vi "LV_multiports_multiservers.vi"() -> ()   [LabVIEW 2020]
panel:
  out "2nd port":string
  out "1st port":string
  in  "Open Multi Ports":bool
  in  "Send Test Img":bool
  in  "h":i32=10 min=1 max=5000 step=1
  in  "w":i32=1 min=1 max=5000 step=1
  out "Elaps ms":u32
  in  "Send Image":bool
  out "Path to Python script":path
  in  "Stop":bool
  out "Answer":string
  in  "Ping":bool
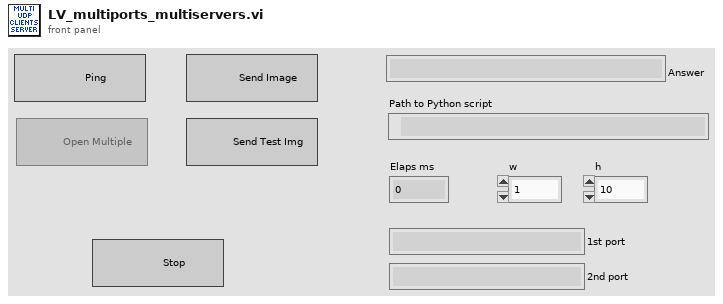
[diagram p1: front panel]
types:
  T1 = enum8{"Enabled", "Disabled", "Disabled and Grayed Out"}
  T2 = typedef "Image Type" = u32
  T3 = typedef "IMAQ Image.ctl" = refnum<image>
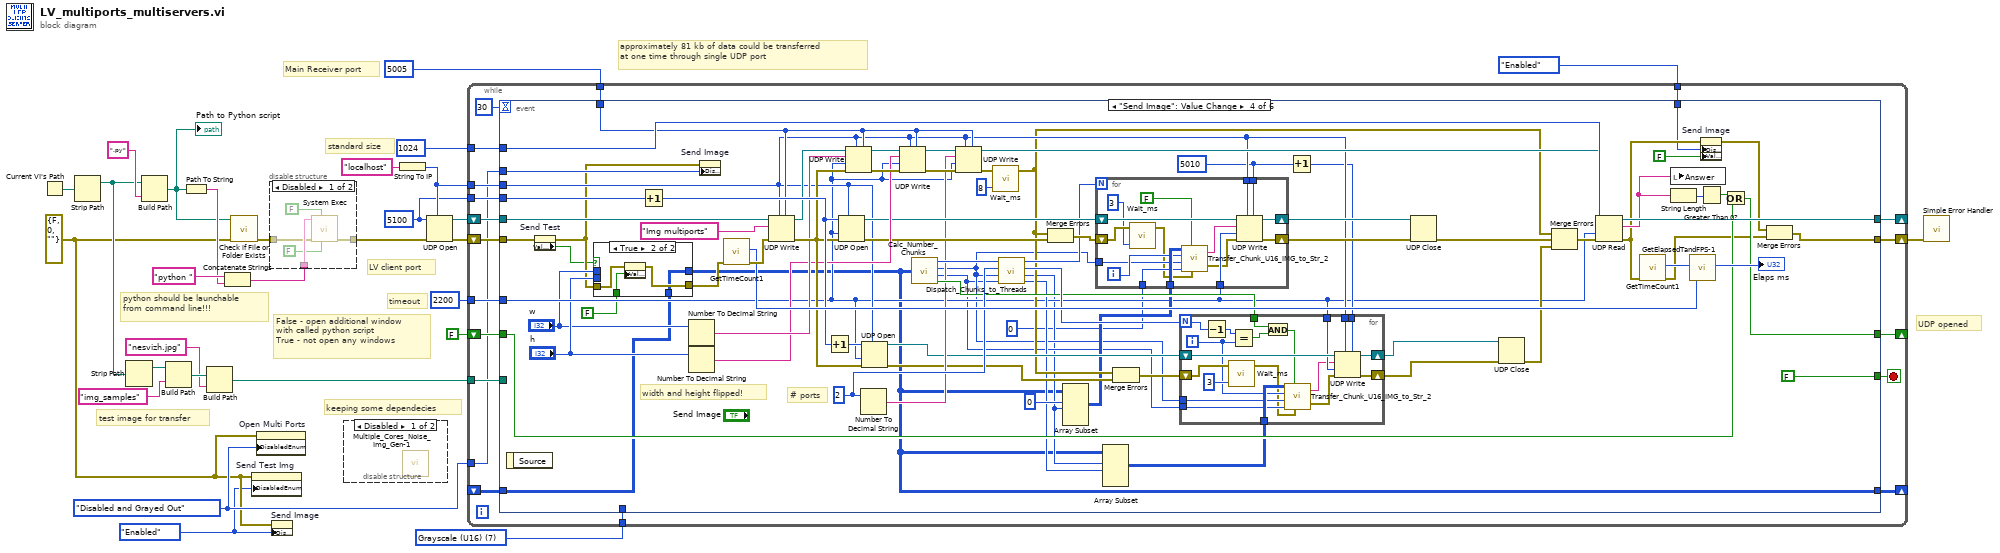
[diagram p0: block diagram]
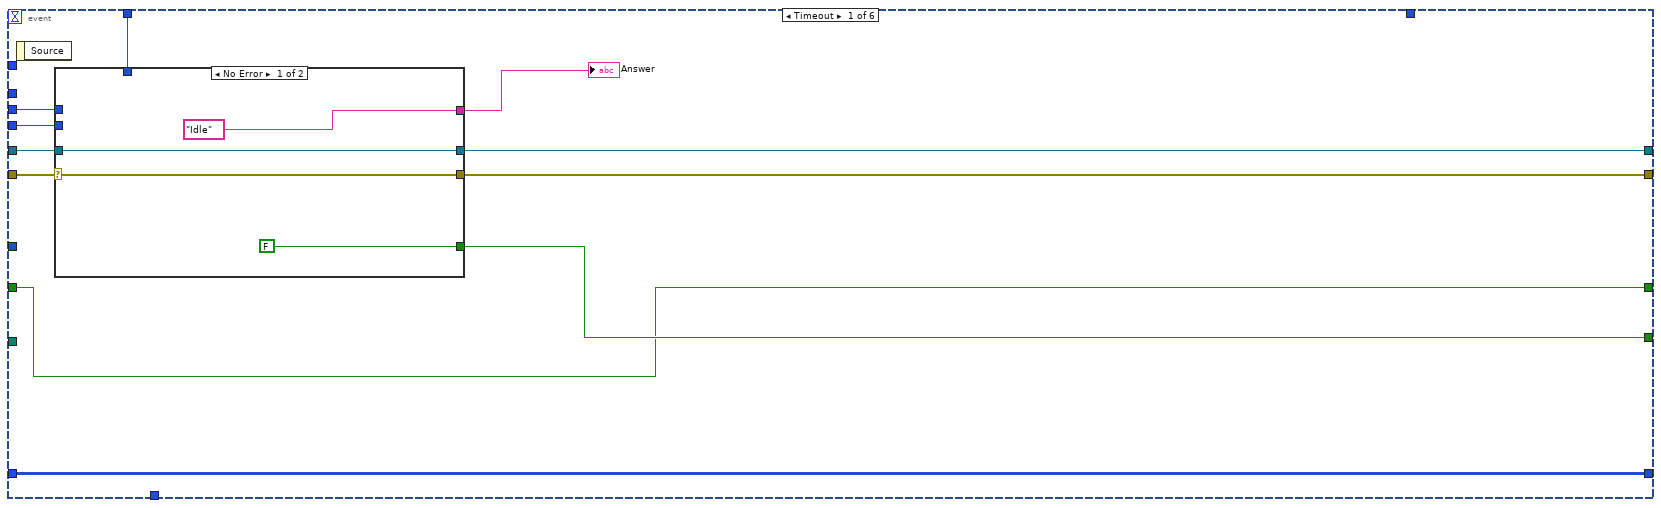
[diagram p4: hidden frame]
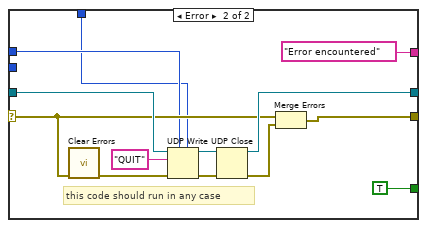
[diagram p5: hidden frame]
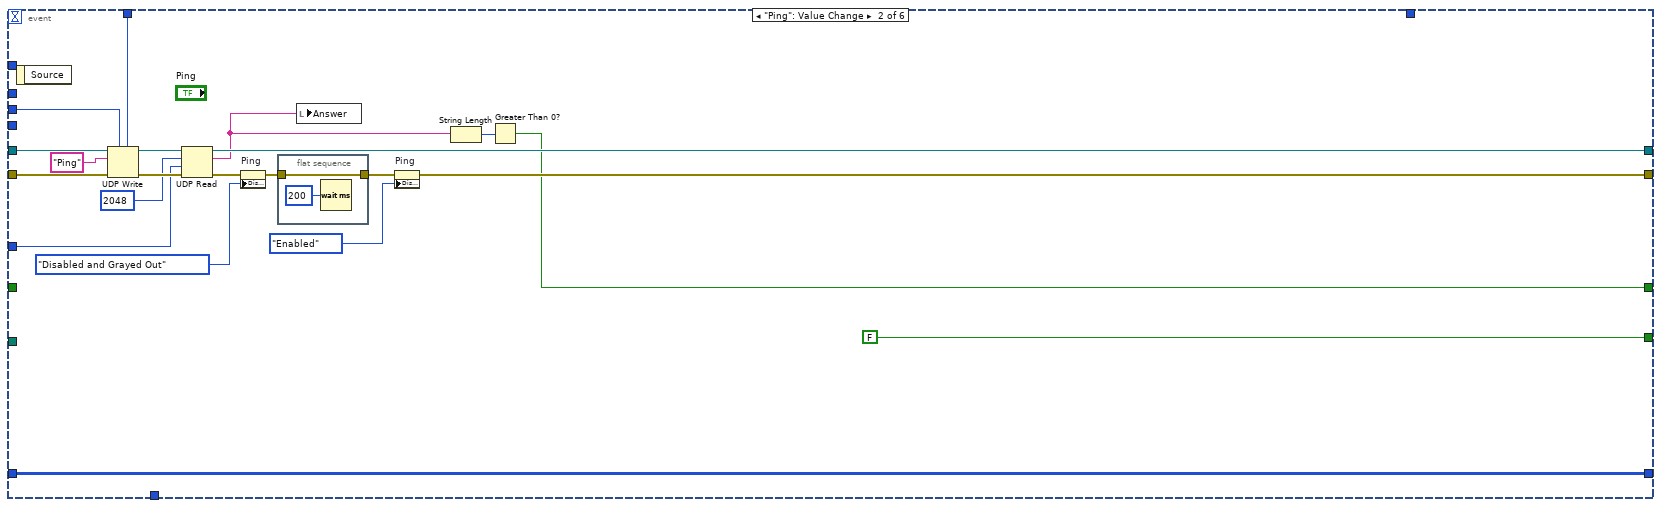
[diagram p6: hidden frame]
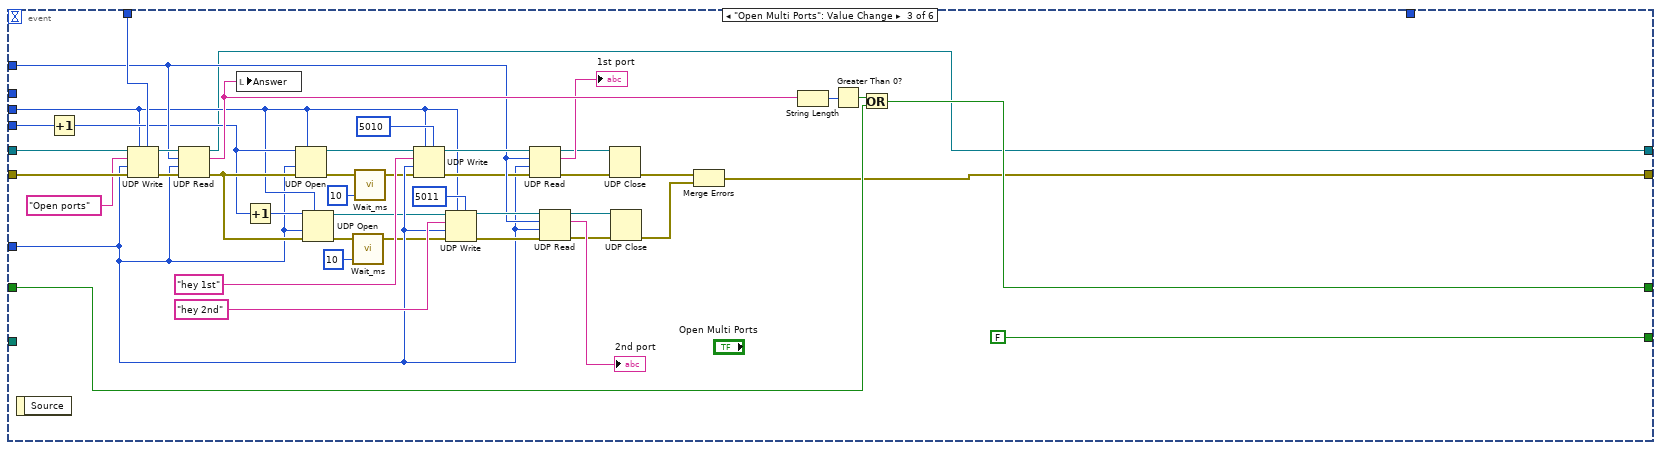
[diagram p7: hidden frame]
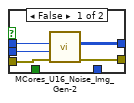
[diagram p8: hidden frame]
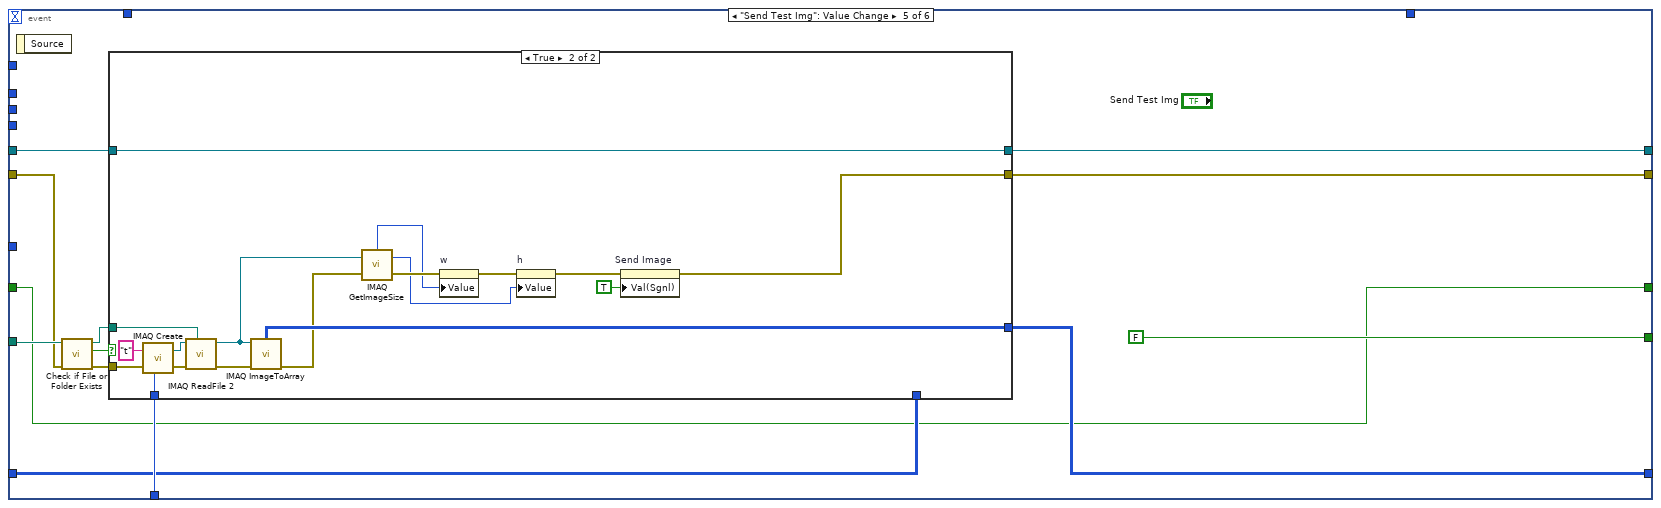
[diagram p9: hidden frame]
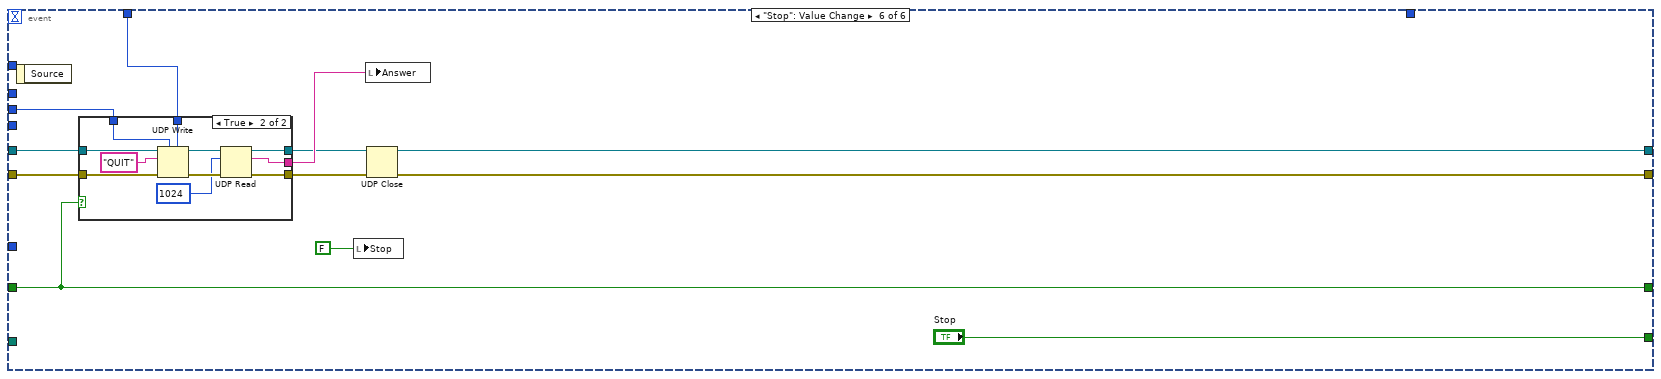
[diagram p11: hidden frame]
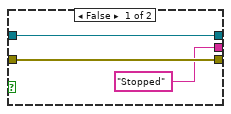
[diagram p12: hidden frame]
diagram:
  w1 = T1."Enabled" ("Disabled")
  w4 = T1."Disabled and Grayed Out" ("Disabled")
  w7 = T2 7 items=["Grayscale (U8)", "Grayscale (I16)", "Grayscale (SGL)", "Complex (CSG)", "RGB (U32)", "HSL (U32)", "RGB (U64)", "Grayscale (U16)"] ("Image Type")
  w16 = u16 5100 ("remote port or service name")
  w2 = errorcluster {"status"=FALSE, "code"=0, "source"=""} ("error in (no error)")
  # "approximately 81 kb of data could be transferred \nat one time through single UDP port"
  # "standard size"
  # "UDP opened"
  # "test image for transfer"
  # "keeping some dependecies"
  # "timeout"
  # "Main Receiver port"
  # "LV client port"
  # "False - open additional window\nwith called python script\nTrue - not open any windows"
  # "python should be launchable \nfrom command line!!!"
  n1 = Current VI's Path() -> (path=w28:path)
  n2 = Strip Path(path=w28) -> (stripped path=w13:path)  [unwired: 1 out]
  n3 = Strip Path(path=w13) -> (stripped path=w12:path)  [unwired: 1 out]
  n4 = Build Path(base path=w13, name or relative path=".py" ("string")) -> (appended path=w23:path)
  "Path to Python script" <- w23
  n5 = Build Path(base path=w12, name or relative path="img_samples" ("string")) -> (appended path=w10:path)
  n6 = Path To String(path=w23) -> (string=w24:string)
  n7 = Build Path(base path=w10, name or relative path="nesvizh.jpg" ("string")) -> (appended path=w8:path)
  n8 = Concatenate Strings("python " ("command line"), w24) -> (w26:string)
  n9 = call <vilib>:"Check if File or Folder Exists.vi"("error in (no error)"=w2, "path"=w23) -> ("error out"=w22:errorcluster)  [unwired: 7 in, 2 out]
  n10 = property on="Send Test Img" class="Bool (strict)"(error in=w2, "DisabledEnum"=w1) -> ()  [unwired: 1 in, 2 out]
  n11 = property on="Open Multi Ports" class="Bool"(error in=w2, "DisabledEnum"=w4) -> ()  [unwired: 1 in, 2 out]
  n12 = disable-structure shown="Disabled" {
    disable-tunnel: w26 -> [w34 _]
    disable-tunnel: [w33 w35] -> w21
    disable-tunnel: w22 -> [w31 w35]
    frame Disabled {
      n13 = call <vilib>:"System Exec.vi"("run minimized? (F)"=FALSE, "wait until completion? (T)"=FALSE, "error in (no error)"=w31, "command line"=w34) -> ("error out"=w33:errorcluster)  [unwired: 4 in, 3 out]
    }
    frame Enabled {
    }
  }
  n14 = property on="Send Image" class="Bool (strict)"(error in=w2, "DisabledEnum"=w1) -> ()  [unwired: 1 in, 2 out]
  n15 = disable-structure shown="Disabled" {
    frame Disabled {
      n16 = call "Multiple_Cores_Noise_Img_Gen-1.vi"() -> ()  [unwired: 10 in, 2 out]
    }
    frame Enabled {
    }
  }
  n17 = String To IP(1:"localhost" ("address")) -> (0:w17:u32)
  n18 = UDP Open(7:w17, 8:w21, 11:w16) -> (port=w19:refnum<k16>, 0:w20:errorcluster)  [unwired: 2 in, 1 out]
  n19 = while {
    shift-right: [w51] -> _
    shift-left: w19 -> [w52]
    shift-right: [w49] -> w29
    shift-left: w20 -> [w53]
    tunnel: w17 -> [w47]
    tunnel: w16 -> [w48]
    tunnel: u16 5005 ("remote port or service name") -> [w46]
    tunnel: 2200 -> [w45]
    tunnel: w8 -> [w44]
    tunnel: w7 -> [w43]
    shift-right: [w41] -> _
    shift-left: FALSE -> [w42]
    tunnel: 1024 -> [w40]
    tunnel: w4 -> [w39]
    tunnel: T1."Enabled" ("Disabled") -> [w38]
    shift-right: [w37] -> _
    shift-left: _ -> [w36]
    stop <- w50 stop-if-true
    n20 = event shown="[3] \"Send Image\": Value Change" {
      selector: _ -> [_ _ _ _ _ _]
      dyn-events: _ -> [_ _ _ _ _ _]
      timeout: 30 -> [_ _ _ _ _ _]
      tunnel: [w61 FALSE ("Stop") FALSE ("Stop") FALSE ("Stop") FALSE ("Stop") "Stop"] -> w50
      tunnel: w53 -> [w65 w97 w150 w155 w283 w313]
      tunnel: w52 -> [w64 w96 w148 w226 w278 w314]
      tunnel: [w63 w92 w118 w224 w276 w315] -> w51
      tunnel: [w62 w99 w130 w160 w277 w316] -> w49
      tunnel: w48 -> [w59 _ w126 w214 _ _]
      tunnel: w47 -> [w58 w89 w121 w186 _ w309]
      tunnel: w46 -> [w57 w88 w147 w198 _ w308]
      tunnel: w45 -> [_ w87 w120 w171 _ _]
      tunnel: w44 -> [_ _ _ _ w284 _]
      tunnel: w43 -> [_ _ _ _ w279 _]
      tunnel: w42 -> [w56 _ w137 w216 w273 w307]
      tunnel: [w56 w84 w136 w215 w273 w307] -> w41
      tunnel: w40 -> [_ _ w133 w213 _ _]
      tunnel: w39 -> [_ _ _ w164 _ _]
      tunnel: w38 -> [_ _ _ w162 _ _]
      tunnel: [w55 w83 _ w157 w275 _] -> w37
      tunnel: w36 -> [w55 w83 _ w151 w274 _]
      event Timeout {
        n21 = event-data() -> ()  [unwired: 1 in, 1 out]
        n22 = case shown="No Error" w65 {
          selector: w65 -> [w68 w77]
          tunnel: [w69 w80] -> w63
          tunnel: w64 -> [w69 w79]
          tunnel: [w68 w78] -> w62
          tunnel: [FALSE ("Stop") TRUE ("Stop")] -> w61
          tunnel: ["Idle" ("Answer") "Error encountered" ("Answer")] -> w60
          tunnel: w59 -> [_ _]
          tunnel: w58 -> [_ w76]
          tunnel: w57 -> [_ w75]
          frame No Error {
          }
          frame Error {
            # "this code should run in any case"
            n23 = call <vilib>:"Clear Errors.vi"("error in (no error)"=w77) -> ("error out"=w74:errorcluster)  [unwired: 5 in, 1 out]
            n24 = UDP Write(address=w76, port or service name=w75, connection ID=w79, data in="QUIT", 8:w74) -> (error out=w73:errorcluster, 3:w71:refnum<k16>)  [unwired: 1 in]
            n25 = UDP Close(connection ID=w71, 8:w73) -> (connection ID out=w80:refnum<k16>, error out=w70:errorcluster)
            n26 = Merge Errors(w77, w70) -> (w78:errorcluster)
          }
        }
        "Answer" <- w60
      }
      event "Ping": Value Change {
        n27 = event-data() -> ()  [unwired: 1 in, 1 out]
        n28 = UDP Write(address=w89, port or service name=w88, connection ID=w96, data in="Ping", 8:w97) -> (error out=w94:errorcluster, 3:w93:refnum<k16>)  [unwired: 1 in]
        n29 = UDP Read(connection ID=w93, max size (548)=2048 ("bytes to read"), timeout ms (25000)=w87, 8:w94) -> (data out=w86:string, error out=w91:errorcluster, 3:w92:refnum<k16>)  [unwired: 2 out]
        n30 = property on="Ping" class="Bool"(error in=w91, "DisabledEnum"=T1."Disabled and Grayed Out" ("Disabled")) -> (error out=w102:errorcluster)  [unwired: 1 in, 1 out]
        n31 = flat-sequence {
          tunnel: w102 -> [w104]
          tunnel: [w104] -> w100
          frame #0 {
            n32 = Wait (ms)(milliseconds to wait=u32 200) -> ()  [unwired: 1 out]
          }
        }
        n33 = local write "Answer"(w86) -> ()
        n34 = property on="Ping" class="Bool"(error in=w100, "DisabledEnum"=T1."Enabled" ("Disabled")) -> (error out=w99:errorcluster)  [unwired: 1 in, 1 out]
        n35 = String Length(string=w86) -> (length=w85:i32)
        n36 = Greater Than 0?(x=w85) -> (x > 0?=w84:bool)
      }
      event "Open Multi Ports": Value Change {
        n37 = event-data() -> ()  [unwired: 1 in, 1 out]
        n38 = Increment(x=w126) -> (x+1=w123:u16)
        n39 = UDP Write(address=w121, port or service name=w147, connection ID=w148, data in="Open ports", 8:w150, 9:w120) -> (error out=w146:errorcluster, 3:w145:refnum<k16>)
        n40 = UDP Read(connection ID=w145, max size (548)=w133, timeout ms (25000)=w120, 8:w146) -> (data out=w138:string, error out=w124:errorcluster, 3:w118:refnum<k16>)  [unwired: 2 out]
        n41 = local write "Answer"(w138) -> ()
        n42 = Increment(x=w123) -> (x+1=w122:u16)
        n43 = UDP Open(7:w121, 8:w124, 9:w120, 11:w123) -> (port=w125:refnum<k16>, 0:w111:errorcluster)  [unwired: 1 in, 1 out]
        n44 = UDP Open(7:w121, 8:w124, 9:w120, 11:w122) -> (port=w119:refnum<k16>, 0:w108:errorcluster)  [unwired: 1 in, 1 out]
        n45 = call "Wait_ms.vi"("[IN] Suspend ms"=u32 10, "error IN"=w108) -> ("error OUT"=w107:errorcluster)  [unwired: 3 in]
        n46 = call "Wait_ms.vi"("[IN] Suspend ms"=u32 10, "error IN"=w111) -> ("error OUT"=w110:errorcluster)  [unwired: 3 in]
        n47 = UDP Write(address=w121, port or service name=u16 5010, connection ID=w125, data in="hey 1st", 8:w110, 9:w120) -> (error out=w128:errorcluster, 3:w135:refnum<k16>)
        n48 = UDP Write(address=w121, port or service name=u16 5011, connection ID=w119, data in="hey 2nd", 8:w107, 9:w120) -> (error out=w127:errorcluster, 3:w134:refnum<k16>)
        n49 = UDP Read(connection ID=w135, max size (548)=w133, timeout ms (25000)=w120, 8:w128) -> (data out=→"1st port":string, error out=w117:errorcluster, 3:w116:refnum<k16>)  [unwired: 2 out]
        n50 = UDP Read(connection ID=w134, max size (548)=w133, timeout ms (25000)=w120, 8:w127) -> (data out=→"2nd port":string, error out=w114:errorcluster, 3:w115:refnum<k16>)  [unwired: 2 out]
        n51 = UDP Close(connection ID=w116, 8:w117) -> (error out=w113:errorcluster)  [unwired: 1 out]
        n52 = UDP Close(connection ID=w115, 8:w114) -> (error out=w112:errorcluster)  [unwired: 1 out]
        n53 = Merge Errors(w113, w112) -> (w130:errorcluster)
        n54 = String Length(string=w138) -> (length=w140:i32)
        n55 = Greater Than 0?(x=w140) -> (x > 0?=w139:bool)
        n56 = Or(x=w139, y=w137) -> (x .or. y?=w136:bool)
      }
      event "Send Image": Value Change {
        w185 = u16 5010 ("remote port or service name")
        w187 = 2
        # "# ports"
        # "width and height flipped!"
        n57 = event-data() -> ()  [unwired: 1 in, 1 out]
        n58 = property on="Send Test" class="Bool (strict)"(error in=w155) -> (error out=w154:errorcluster, "Value"=w153:bool)  [unwired: 1 in, 1 out]
        n59 = case shown="True" w153 {
          tunnel: "h" -> [w232 _]
          tunnel: "w" -> [w231 _]
          tunnel: [w230 w234] -> w165
          tunnel: w154 -> [w229 w236]
          tunnel: [w228 w233] -> w157
          tunnel: FALSE ("Send Test Img") -> [_ w235]
          tunnel: w151 -> [_ w233]
          frame False {
            n60 = call "MCores_U16_Noise_Img_Gen-2.vi"("error IN"=w229, "[IN] Width"=w232, "[IN] Height"=w231) -> ("error OUT"=w230:errorcluster, "[OUT] U16 Pixel Img"=w228:u16[][])  [unwired: 7 in]
          }
          frame True {
            n61 = property on="Send Test Img" class="Bool (strict)"(error in=w236, "Value"=w235) -> (error out=w234:errorcluster)  [unwired: 1 in, 1 out]
          }
        }
        n62 = Increment(x=w214) -> (x+1=w212:u16)
        n63 = Number To Decimal String(number="w") -> (decimal integer string=w208:string)  [unwired: 1 in]
        n64 = Number To Decimal String(number="h") -> (decimal integer string=w205:string)  [unwired: 1 in]
        n65 = property on="Send Image" class="Bool (strict)"(error in=w154, "DisabledEnum"=w164) -> ()  [unwired: 1 in, 2 out]
        n66 = call "GetTimeCount1.vi"("error IN"=w165) -> ("error OUT"=w223:errorcluster, "[OUT] Timer Count"=w221:u32)  [unwired: 9 in]
        n67 = UDP Write(address=w186, port or service name=w198, connection ID=w226, data in="Img multiports", 8:w223) -> (error out=w210:errorcluster, 3:w209:refnum<k16>)  [unwired: 1 in]
        n68 = Increment(x=w212) -> (x+1=w211:u16)
        n69 = UDP Open(7:w186, 8:w210, 9:w171, 11:w212) -> (port=w195:refnum<k16>, 0:w190:errorcluster)  [unwired: 1 in, 1 out]
        n70 = UDP Write(address=w186, port or service name=w198, connection ID=w209, data in=w208, 8:w210, 9:w171) -> (error out=w207:errorcluster, 3:w206:refnum<k16>)
        n71 = Number To Decimal String(number=w187) -> (decimal integer string=w181:string)  [unwired: 1 in]
        n72 = UDP Open(7:w186, 8:w210, 9:w171, 11:w211) -> (port=w180:refnum<k16>, 0:w179:errorcluster)  [unwired: 1 in, 1 out]
        n73 = UDP Write(address=w186, port or service name=w198, connection ID=w206, data in=w205, 8:w207, 9:w171) -> (error out=w200:errorcluster, 3:w199:refnum<k16>)
        n74 = call "Calc_Number_Chunks.vi"("[IN] U16 Pixel Img"=w157) -> ("[OUT] Number of chunks"=w201:i32, "[OUT] # rows single transfer"=w170:i32, "[OUT] # rows last transfer"=w169:i32, "[OUT] Not-equal last transfer"=w182:bool)
        n75 = UDP Write(address=w186, port or service name=w198, connection ID=w199, data in=w181, 8:w200, 9:w171) -> (error out=w191:errorcluster, 3:w197:refnum<k16>)
        n76 = call "Wait_ms.vi"("[IN] Suspend ms"=u32 8, "error IN"=w191) -> ("error OUT"=w178:errorcluster)  [unwired: 3 in]
        n77 = call "Dispatch_Chunks_to_Threads.vi"("[IN] # rows last transfer"=w169, "[IN] # rows single transfer"=w170, "[IN] Number of threads"=w187, "[IN] Number of chunks"=w201) -> ("[OUT] Remained rows last transfer"=w172:i32, "[OUT] Rows of img for port"=w168:i32, "[OUT] Dispatched lastly"=w183:i32, "[OUT] Dispatched chunks"=w188:i32)
        n78 = Merge Errors(w178, w190) -> (w189:errorcluster)
        n79 = Array Subset(array=w157, index (row)=0 ("index"), length (row)=w168) -> (w176:u16[][])  [unwired: 2 in]
        n80 = for {
          N: w188 -> [_]
          shift-right: [w272] -> w193
          shift-left: w189 -> [w266]
          shift-right: [w271] -> w194
          shift-left: w195 -> [w270]
          tunnel: w186 -> [w269]
          tunnel: w185 -> [w268]
          tunnel: w170 -> [w259]
          tunnel: w176 -> [w261]
          tunnel: w171 -> [w267]
          tunnel: 0 ("[IN] # rows last transfer") -> [w258]
          i -> [w260]
          n81 = call "Wait_ms.vi"("[IN] Suspend ms"=u32 3, "error IN"=w266) -> ("error OUT"=w257:errorcluster)  [unwired: 3 in]
          n82 = call "Transfer_Chunk_U16_IMG_to_Str_2.vi"("error IN"=w257, "[IN] Use remained rows"=FALSE, "[IN] # rows last transfer"=w258, "[IN] # rows single transfer"=w259, "[IN] # of chunk"=w260, "[IN] U16 Pixel Img"=w261) -> ("error OUT"=w262:errorcluster, "[OUT] Converted String"=w263:string)
          n83 = UDP Write(address=w269, port or service name=w268, connection ID=w270, data in=w263, 8:w262, 9:w267) -> (error out=w272:errorcluster, 3:w271:refnum<k16>)
        }
        n84 = Array Subset(array=w157, index (row)=w168, length (row)=w172) -> (w175:u16[][])  [unwired: 2 in]
        n85 = Merge Errors(w178, w179) -> (w177:errorcluster)
        n86 = Increment(x=w185) -> (x+1=w184:u16)
        n87 = for {
          N: w183 -> [w256]
          shift-right: [w252] -> w173
          shift-left: w177 -> [w246]
          tunnel: w175 -> [w243]
          tunnel: w170 -> [w241]
          tunnel: w169 -> [w240]
          shift-right: [w251] -> w174
          shift-left: w180 -> [w250]
          tunnel: w182 -> [w254]
          tunnel: w186 -> [w249]
          tunnel: w184 -> [w248]
          tunnel: w171 -> [w247]
          i -> [w242]
          n88 = Decrement(x=w256) -> (x-1=w255:i32)
          n89 = call "Wait_ms.vi"("[IN] Suspend ms"=u32 3, "error IN"=w246) -> ("error OUT"=w239:errorcluster)  [unwired: 3 in]
          n90 = Equal?(x=w255, y=w242) -> (x = y?=w253:bool)
          n91 = And(x=w254, y=w253) -> (x .and. y?=w244:bool)
          n92 = call "Transfer_Chunk_U16_IMG_to_Str_2.vi"("error IN"=w239, "[IN] Use remained rows"=w244, "[IN] # rows last transfer"=w240, "[IN] # rows single transfer"=w241, "[IN] # of chunk"=w242, "[IN] U16 Pixel Img"=w243) -> ("error OUT"=w237:errorcluster, "[OUT] Converted String"=w238:string)
          n93 = UDP Write(address=w249, port or service name=w248, connection ID=w250, data in=w238, 8:w237, 9:w247) -> (error out=w252:errorcluster, 3:w251:refnum<k16>)
        }
        n94 = UDP Close(connection ID=w194, 8:w193) -> (error out=w204:errorcluster)  [unwired: 1 out]
        n95 = UDP Close(connection ID=w174, 8:w173) -> (error out=w202:errorcluster)  [unwired: 1 out]
        n96 = Merge Errors(w178, w204, w202) -> (w203:errorcluster)
        n97 = UDP Read(connection ID=w197, max size (548)=w213, timeout ms (25000)=w171, 8:w203) -> (data out=w218:string, error out=w163:errorcluster, 3:w224:refnum<k16>)  [unwired: 2 out]
        n98 = call "GetTimeCount1.vi"("error IN"=w163) -> ("error OUT"=w159:errorcluster, "[OUT] Timer Count"=w222:u32)  [unwired: 9 in]
        n99 = local write "Answer"(w218) -> ()
        n100 = String Length(string=w218) -> (length=w219:i32)
        n101 = call "GetElapsedTandFPS-1.vi"("[IN] Timer Count Before ALL [ms]"=w221, "[IN] Timer Count After ALL [ms]"=w222) -> ("[OUT] Elapsed time [ms]"=→"Elaps ms":u32)  [unwired: 3 in, 2 out]
        n102 = Greater Than 0?(x=w219) -> (x > 0?=w217:bool)
        n103 = property on="Send Image" class="Bool (strict)"(error in=w163, "DisabledEnum"=w162, "Value"=FALSE ("Send Image")) -> (error out=w161:errorcluster)  [unwired: 1 in, 1 out]
        n104 = Or(x=w217, y=w216) -> (x .or. y?=w215:bool)
        n105 = Merge Errors(w161, w159) -> (w160:errorcluster)
      }
      event "Send Test Img": Value Change {
        n106 = event-data() -> ()  [unwired: 1 in, 1 out]
        n107 = call <vilib>:"Check if File or Folder Exists.vi"("error in (no error)"=w283, "path"=w284) -> ("error out"=w282:errorcluster, "file or folder exists?"=w281:bool, "dup path"=w280:path)  [unwired: 7 in]
        n108 = case shown="True" w281 {
          tunnel: w282 -> [w287 w306]
          tunnel: w280 -> [_ w301]
          tunnel: w279 -> [_ w305]
          tunnel: w278 -> [w288 w293]
          tunnel: [w287 w291] -> w277
          tunnel: [w288 w293] -> w276
          tunnel: [w286 w296] -> w275
          tunnel: w274 -> [w286 _]
          frame False {
          }
          frame True {
            n109 = call "IMAQ Create"("Image Name"="t", "Image Type"=w305, "error in (no error)"=w306) -> ("New Image"=w302:T3, "error out"=w303:errorcluster)  [unwired: 2 in]
            n110 = call "IMAQ ReadFile 2"("File Path"=w301, "error in (no error)"=w303, "Image"=w302) -> ("error out"=w299:errorcluster, "Image Out"=w300:T3)  [unwired: 4 in, 3 out]
            n111 = call "IMAQ ImageToArray"("error in (no error)"=w299, "Image"=w300) -> ("error out"=w295:errorcluster, "Image Pixels (U8)"=w296:u8[][])  [unwired: 2 in, 3 out]
            n112 = call "IMAQ GetImageSize"("Image"=w300, "error in (no error)"=w295) -> ("Y Resolution"=w289:i32, "X Resolution"=w290:i32, "error out"=w298:errorcluster)  [unwired: 2 in]
            n113 = property on="w" class="DigNum (strict)"(error in=w298, "Value"=w290) -> (error out=w297:errorcluster)  [unwired: 1 in, 1 out]
            n114 = property on="h" class="DigNum (strict)"(error in=w297, "Value"=w289) -> (error out=w294:errorcluster)  [unwired: 1 in, 1 out]
            n115 = property on="Send Image" class="Bool (strict)"(error in=w294, "Val(Sgnl)"=TRUE ("Value (Signaling)")) -> (error out=w291:errorcluster)  [unwired: 1 in, 1 out]
          }
        }
      }
      event "Stop": Value Change {
        n116 = event-data() -> ()  [unwired: 1 in, 1 out]
        n117 = case shown="True" w307 {
          tunnel: w314 -> [w321 w332]
          tunnel: w313 -> [w320 w331]
          tunnel: [w320 w327] -> w312
          tunnel: ["Stopped" ("data out") w326] -> w311
          tunnel: [w321 w325] -> w310
          tunnel: w309 -> [_ w323]
          tunnel: w308 -> [_ w322]
          frame False {
          }
          frame True {
            n118 = UDP Write(address=w323, port or service name=w322, connection ID=w332, data in="QUIT", 8:w331) -> (error out=w328:errorcluster, 3:w329:refnum<k16>)  [unwired: 1 in]
            n119 = UDP Read(connection ID=w329, max size (548)=1024 ("bytes to read"), 8:w328) -> (data out=w326:string, error out=w327:errorcluster, 3:w325:refnum<k16>)  [unwired: 1 in, 2 out]
          }
        }
        n120 = local write "Stop"(FALSE ("Stop")) -> ()
        n121 = local write "Answer"(w311) -> ()
        n122 = UDP Close(connection ID=w310, 8:w312) -> (connection ID out=w315:refnum<k16>, error out=w316:errorcluster)
      }
    }
  }
  n123 = call <vilib>:"Simple Error Handler.vi"("error in (no error)"=w29) -> ()  [unwired: 4 in, 5 out]
